vi "Check mtcdt firmware.vi"(6 "VISA resource name":refnum<visa-resource-name>="COM5", 7 "Passed so far":bool, 8 "error in (no error)":errorcluster) -> (0 "error out":errorcluster, 2 "Response":string, 3 "Keyword found index":i32, 4 "VISA Refnum out":refnum<visa-resource-name>, 5 "Passed?":bool)   [LabVIEW 2024]
panel:
  out "Keyword found":string
  in  "Wait for keywords":string[](array[string])=["5.3.26", "5.3.31", "6.0.2", "6.3.0"]
  in  "write buffer":string="cat /etc/issue.net\n"
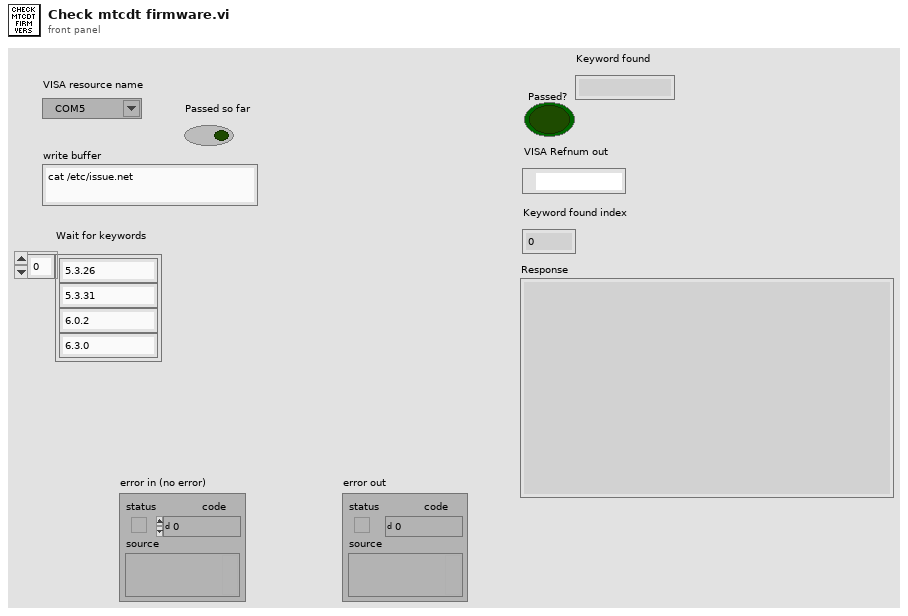
[diagram p1: front panel]
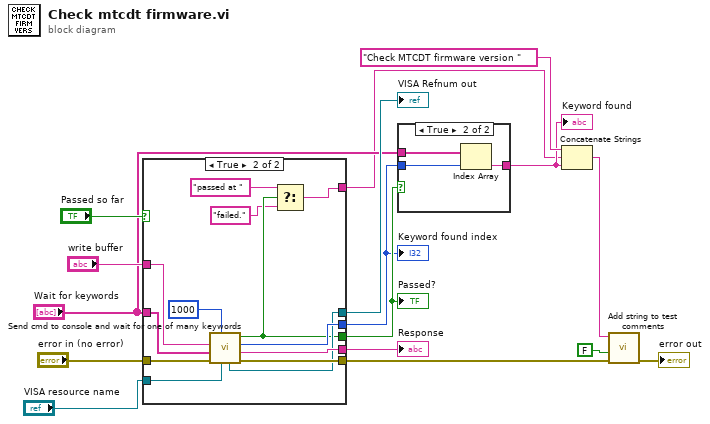
[diagram p0: block diagram]
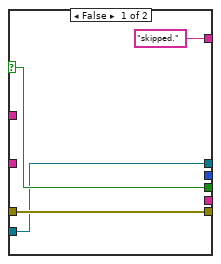
[diagram p3: hidden frame]
diagram:
  n1 = case shown="True" "Passed so far" {
    selector: "Passed so far" -> [w20 _]
    tunnel: "error in (no error)" -> [w19 w33]
    tunnel: [w19 w32] -> w7
    tunnel: "VISA resource name" -> [w18 w26]
    tunnel: "write buffer" -> [_ w31]
    tunnel: "Wait for keywords" -> [_ w30]
    tunnel: [w20 w24] -> w5
    tunnel: [_ w28] -> w3
    tunnel: [_ w27] -> w13
    tunnel: [w18 w25] -> w11
    tunnel: ["skipped." w21] -> w1
    frame False {
    }
    frame True {
      n2 = call "Send cmd to console and wait for one of many keywords.vi"("VISA resource name"=w26, "Timeout (1000 mSecs)"=u32 1000 ("Timeout (mSecs)"), "error in (no error)"=w33, "Wait for keywords"=w30, "write buffer"=w31) -> ("error out"=w32:errorcluster, "Response"=w27:string, "Keyword found index"=w28:i32, "Found key?"=w24:bool, "VISA Refnum out"=w25:refnum<visa-resource-name>)  [unwired: 2 in]
      n3 = Select(t="passed at ", s=w24, f="failed.") -> (s? t:f=w21:string)
    }
  }
  "Passed?" <- w5
  "Keyword found index" <- w3
  "Response" <- w13
  "VISA Refnum out" <- w11
  n4 = case shown="True" w5 {
    tunnel: "Wait for keywords" -> [_ w36]
    tunnel: w3 -> [_ w35]
    tunnel: [_ w34] -> w2
    frame False {
    }
    frame True {
      n5 = Index Array(array=w36, index=w35) -> (element=w34:string)
    }
  }
  "Keyword found" <- w2
  n6 = Concatenate Strings("Check MTCDT firmware version " ("string"), w1, w2) -> (w9:string)
  n7 = call "Add string to test comments.vi"("error in (no error)"=w7, "New Section (y)?"=FALSE, "Comments"=w9) -> ("error out"=→"error out":errorcluster)  [unwired: 7 in, 1 out]
